vi "TCP read to CRLF.vi"(8 "error in":errorcluster, 9 "timeout":i32, 10 "bytes to read":i32, 11 "connection ID":refnum<k5>) -> (0 "error out":errorcluster, 1 "timed out?":bool, 2 "data":u8[](array[numeric]))   [LabVIEW 2013, in "TCP Shared Components.lvlib"]
doc: "This function reads a TCP string from the bus up until a CRLF and checks for errors. It is a wrapper for standard functionality."
uses:
  TCP Shared Components.lvlib
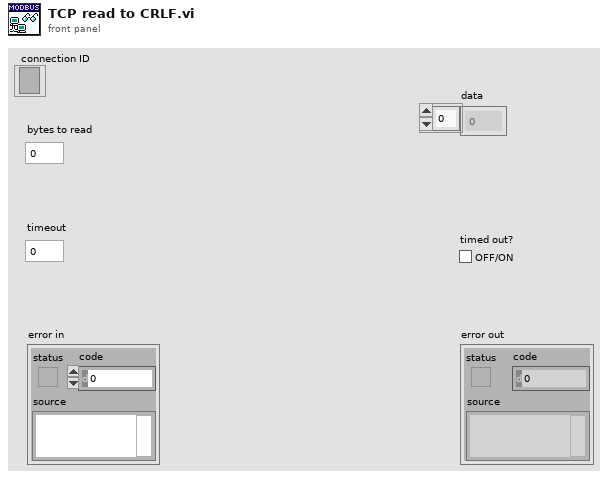
[diagram p1: front panel]
types:
  T1 = enum16{"Standard", "Buffered", "CRLF", "Immediate"}
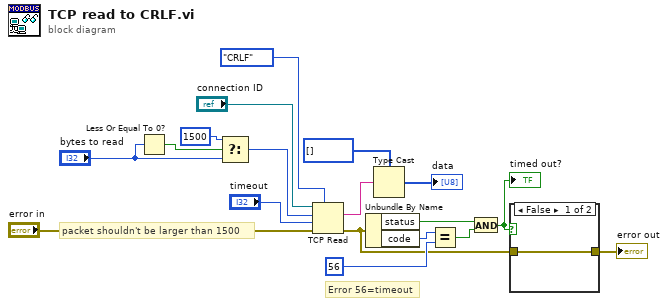
[diagram p0: block diagram]
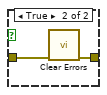
[diagram p2: hidden frame]
diagram:
  # "packet shouldn't be larger than 1500"
  # "Error 56=timeout"
  n1 = Less Or Equal To 0?(x="bytes to read") -> (x <= 0?=w1:bool)
  n2 = Select(t=1500, s=w1, f="bytes to read") -> (s? t:f=w5:i32)
  n3 = TCP Read(connection ID="connection ID", bytes to read=w5, error in (no error)="error in", 7:T1."CRLF" ("mode (standard)"), 9:"timeout") -> (data out=w7:string, error out=w6:errorcluster)  [unwired: 1 out]
  n4 = Unbundle By Name(w6) -> ("status"=w10:bool, "code"=w12:i32)
  n5 = Type Cast(type=u8[] [] ("data"), x=w7) -> (*(type *) &x=→"data":u8[])
  n6 = Equal?(x=w12, y=56) -> (x = y?=w9:bool)
  n7 = And(x=w10, y=w9) -> (x .and. y?=w16:bool)
  "timed out?" <- w16
  n8 = case shown="False" w16 {
    tunnel: w6 -> [w19 w21]
    tunnel: [w19 w20] -> w17
    frame False {
    }
    frame True {
      n9 = call <vilib>:"Clear Errors.vi"("error in (no error)"=w21) -> ("error out"=w20:errorcluster)  [unwired: 6 in]
    }
  }
  "error out" <- w17
